vi "Maximize VI Panel.vi"(7 "Close Reference (T)":bool=TRUE, 8 "error in (no error)":errorcluster, 10 "Method (Maximize on Primary)":T1(ring), 11 "VI Ref (calling VI)":refnum<vi>) -> (0 "error out":errorcluster)   [LabVIEW 2021, in "Panel Movement Center Maximize.lvlib"]
doc: "This VI will maximize a VI to the provided monitor. Optionally pass in the VI Reference to the VI. If no reference is passed in the parent VI will be used.\n\n\n-----\nHooovahh\n(Brian Hoover)"
uses:
  Panel Movement Center Maximize.lvlib
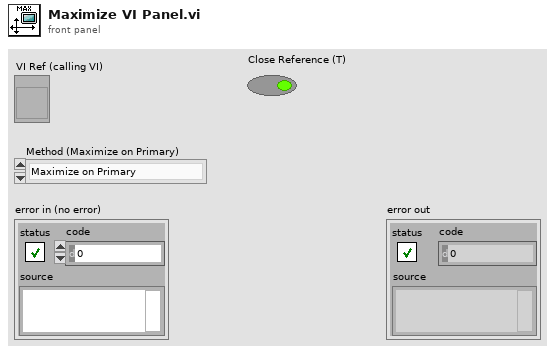
[diagram p1: front panel]
types:
  T1 = enum16{"Maximize on Primary", "Maximize on Secondary", "Maximize on Third", "Maximize on Left", "Maximize on Right", "Maximize Second From Left"}
  T2 = enum32{"Invalid", "Standard", "Closed", "Hidden", "Minimized", "Maximized"}
  T3 = cluster{"Left":i16, "Top":i16, "Right":i16, "Bottom":i16}[]
  T4 = cluster{"Left":i16, "Top":i16, "Right":i16, "Bottom":i16}
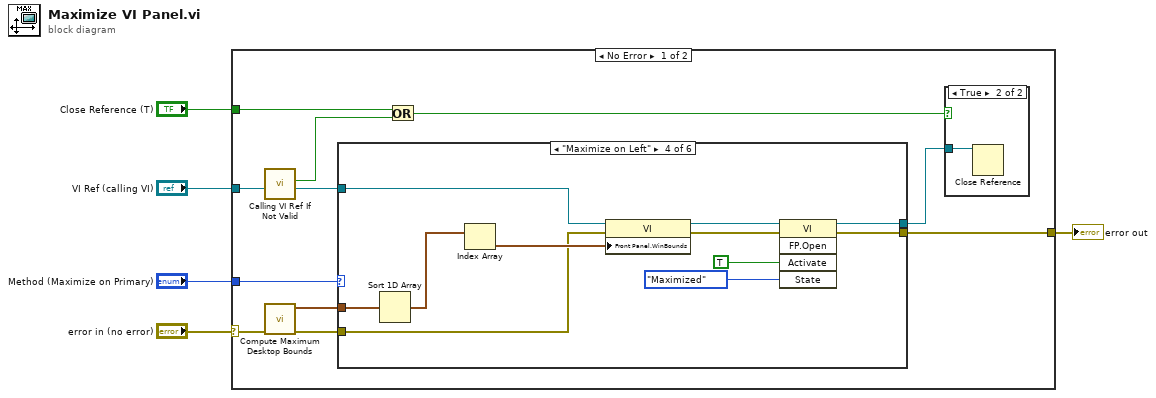
[diagram p0: block diagram]
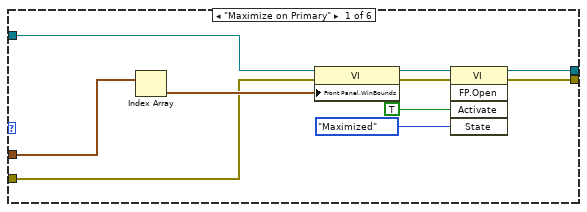
[diagram p3: hidden frame]
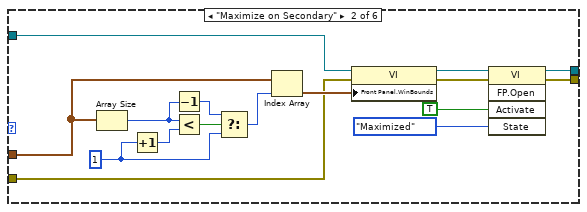
[diagram p4: hidden frame]
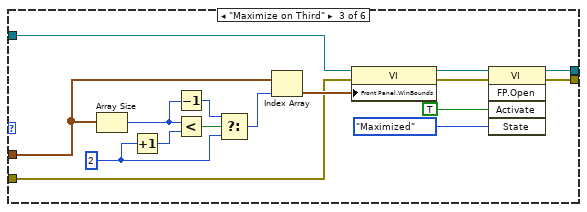
[diagram p5: hidden frame]
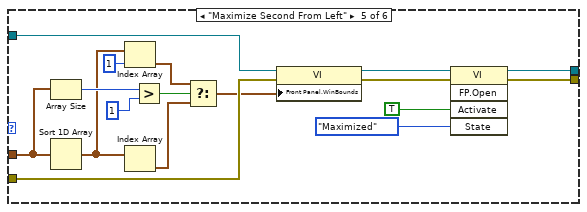
[diagram p6: hidden frame]
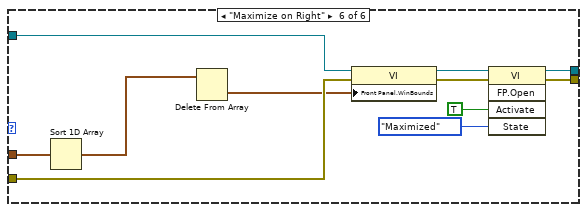
[diagram p7: hidden frame]
diagram:
  n1 = case shown="No Error" "error in (no error)" {
    selector: "error in (no error)" -> [w14 w99]
    tunnel: "VI Ref (calling VI)" -> [w16 _]
    tunnel: "Method (Maximize on Primary)" -> [w15 _]
    tunnel: [w10 w99] -> w2
    tunnel: "Close Reference (T)" -> [w8 _]
    frame No Error {
      n2 = call "Calling VI Ref If Not Valid.vi"("VI Reference"=w16) -> ("Valid VI Ref"=w11:refnum<vi>, "New Reference Opened"=w9:bool)  [unwired: 8 in, 1 out]
      n3 = call "Compute Maximum Desktop Bounds.vi"("error in (no error)"=w14) -> ("error out"=w13:errorcluster, "All Monitor Positions"=w12:T3)  [unwired: 7 in, 2 out]
      n4 = case shown="\"Maximize on Left\"" w15 {
        tunnel: w13 -> [w20 w37 w53 w63 w82 w93]
        tunnel: w12 -> [w23 w34 w50 w66 w78 w90]
        tunnel: w11 -> [w21 w38 w54 w64 w83 w94]
        tunnel: [w19 w36 w52 w62 w81 w92] -> w10
        tunnel: [w18 w35 w51 w61 w80 w91] -> w6
        frame "Maximize on Primary" {
          n5 = Index Array(array=w23) -> (element=w22:T4)  [unwired: 1 in]
          n6 = property class="VI"(reference=w21, error in=w20, "Front Panel.WinBounds"=w22) -> (reference out=w24:refnum<vi>, error out=w25:errorcluster)
          n7 = invoke class="VI" method="FP.Open"(reference=w24, error in=w25, "Activate"=TRUE ("Activate?"), "State"=T2."Maximized") -> (reference out=w18:refnum<vi>, error out=w19:errorcluster)  [unwired: 1 in, 3 out]
        }
        frame "Maximize on Secondary" {
          w32 = 1 ("y")
          n8 = Array Size(array=w34) -> (size(s)=w29:i32)
          n9 = Increment(x=w32) -> (x+1=w30:i32)
          n10 = Decrement(x=w29) -> (x-1=w28:i32)
          n11 = Less?(x=w29, y=w30) -> (x < y?=w33:bool)
          n12 = Select(t=w28, s=w33, f=w32) -> (s? t:f=w31:i32)
          n13 = Index Array(array=w34, index=w31) -> (element=w39:T4)
          n14 = property class="VI"(reference=w38, error in=w37, "Front Panel.WinBounds"=w39) -> (reference out=w40:refnum<vi>, error out=w41:errorcluster)
          n15 = invoke class="VI" method="FP.Open"(reference=w40, error in=w41, "Activate"=TRUE ("Activate?"), "State"=T2."Maximized") -> (reference out=w35:refnum<vi>, error out=w36:errorcluster)  [unwired: 1 in, 3 out]
        }
        frame "Maximize on Third" {
          w48 = 2 ("y")
          n16 = Array Size(array=w50) -> (size(s)=w45:i32)
          n17 = Increment(x=w48) -> (x+1=w46:i32)
          n18 = Decrement(x=w45) -> (x-1=w44:i32)
          n19 = Less?(x=w45, y=w46) -> (x < y?=w49:bool)
          n20 = Select(t=w44, s=w49, f=w48) -> (s? t:f=w47:i32)
          n21 = Index Array(array=w50, index=w47) -> (element=w55:T4)
          n22 = property class="VI"(reference=w54, error in=w53, "Front Panel.WinBounds"=w55) -> (reference out=w56:refnum<vi>, error out=w57:errorcluster)
          n23 = invoke class="VI" method="FP.Open"(reference=w56, error in=w57, "Activate"=TRUE ("Activate?"), "State"=T2."Maximized") -> (reference out=w51:refnum<vi>, error out=w52:errorcluster)  [unwired: 1 in, 3 out]
        }
        frame "Maximize on Left" {
          n24 = Sort 1D Array(array=w66) -> (sorted array=w60:T3)
          n25 = Index Array(array=w60) -> (element=w65:T4)  [unwired: 1 in]
          n26 = property class="VI"(reference=w64, error in=w63, "Front Panel.WinBounds"=w65) -> (reference out=w67:refnum<vi>, error out=w68:errorcluster)
          n27 = invoke class="VI" method="FP.Open"(reference=w67, error in=w68, "Activate"=TRUE ("Activate?"), "State"=T2."Maximized") -> (reference out=w61:refnum<vi>, error out=w62:errorcluster)  [unwired: 1 in, 3 out]
        }
        frame "Maximize Second From Left" {
          n28 = Array Size(array=w78) -> (size(s)=w77:i32)
          n29 = Sort 1D Array(array=w78) -> (sorted array=w76:T3)
          n30 = Index Array(array=w76, index=1) -> (element=w73:T4)
          n31 = Index Array(array=w76) -> (element=w74:T4)  [unwired: 1 in]
          n32 = Greater?(x=w77, y=1 ("x")) -> (0:w75:bool)
          n33 = Select(t=w73, s=w75, f=w74) -> (s? t:f=w72:T4)
          n34 = property class="VI"(reference=w83, error in=w82, "Front Panel.WinBounds"=w72) -> (reference out=w84:refnum<vi>, error out=w85:errorcluster)
          n35 = invoke class="VI" method="FP.Open"(reference=w84, error in=w85, "Activate"=TRUE ("Activate?"), "State"=T2."Maximized") -> (reference out=w80:refnum<vi>, error out=w81:errorcluster)  [unwired: 1 in, 3 out]
        }
        frame "Maximize on Right" {
          n36 = Sort 1D Array(array=w90) -> (sorted array=w89:T3)
          n37 = Delete From Array(array=w89) -> (deleted portion=w88:T4)  [unwired: 2 in, 1 out]
          n38 = property class="VI"(reference=w94, error in=w93, "Front Panel.WinBounds"=w88) -> (reference out=w95:refnum<vi>, error out=w96:errorcluster)
          n39 = invoke class="VI" method="FP.Open"(reference=w95, error in=w96, "Activate"=TRUE ("Activate?"), "State"=T2."Maximized") -> (reference out=w91:refnum<vi>, error out=w92:errorcluster)  [unwired: 1 in, 3 out]
        }
      }
      n40 = Or(x=w8, y=w9) -> (x .or. y?=w7:bool)
      n41 = case shown="True" w7 {
        tunnel: w6 -> [_ w17]
        frame False {
        }
        frame True {
          n42 = Close Reference(reference=w17) -> ()  [unwired: 1 in, 1 out]
        }
      }
    }
    frame Error {
    }
  }
  "error out" <- w2
